vi "Start Sync.vi"(8 "error in":errorcluster, 11 "gRPC Server in":refnum<class "ServiceBase.lvclass">) -> (0 "error out":errorcluster, 3 "gRPC Server out":refnum<class "ServiceBase.lvclass">)   [LabVIEW 2020, in "gRPC-servicer-release.lvlib" / "ServiceBase.lvclass"]
uses:
  gRPC Data Server Engine Windows.llb/ServiceBase.lvclass
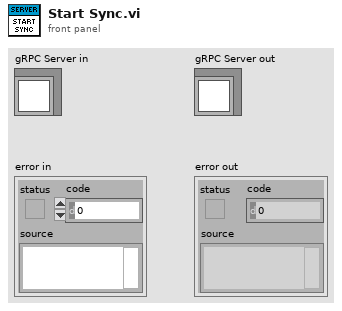
[diagram p1: front panel]
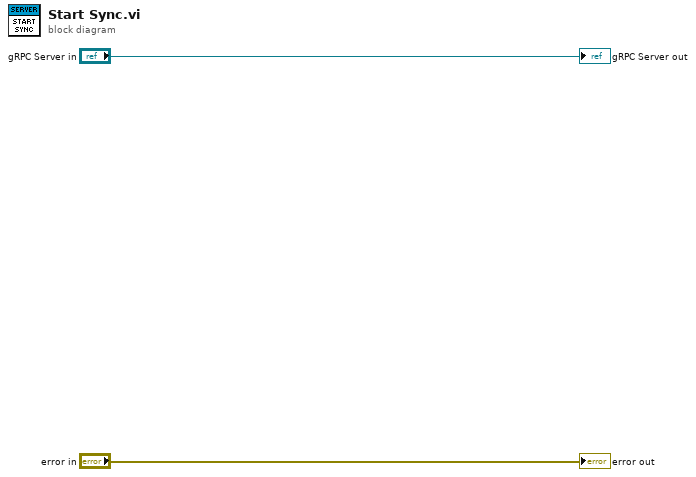
[diagram p0: block diagram]
diagram:
  "error out" <- "error in"
  "gRPC Server out" <- "gRPC Server in"
